vi "Do.vi"(8 "error in (no error)":errorcluster, 10 "Actor in":refnum<class "Actor.lvclass">, 11 "After Launch Init Msg":refnum<class "After Launch Init Msg.lvclass">) -> (0 "error out":errorcluster, 2 "Actor out":refnum<class "Actor.lvclass">)   [LabVIEW 2015, in "CS++BaseActor.lvlib" / "After Launch Init Msg.lvclass"]
doc: "This VI delivers the message to the actor by calling the appropriate method(s) on the actor."
uses:
  After Launch Init Msg.lvclass
  <vilib>/ActorFramework/Actor/Actor.lvclass
  CS++BaseActor/CS++BaseActor.lvclass
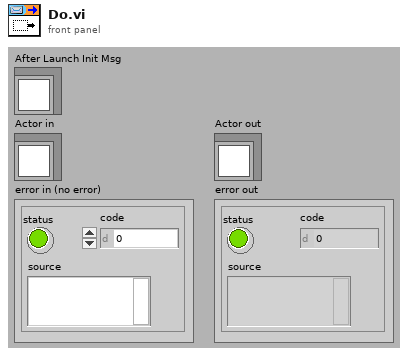
[diagram p1: front panel]
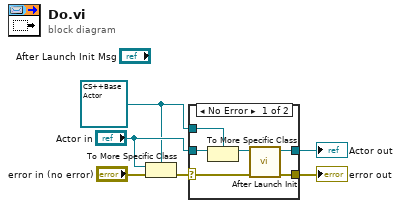
[diagram p0: block diagram]
diagram:
  w1 = refnum<class "CS++BaseActor.lvclass"> refnum ("Actor in")
  n1 = To More Specific Class(target class=w1, reference="Actor in", error in="error in (no error)") -> (error out=w5:errorcluster)  [unwired: 1 out]
  n2 = case shown="No Error" w5 {
    selector: w5 -> [w10 w14]
    tunnel: [w12 w14] -> w4
    tunnel: [w11 w13] -> w3
    tunnel: "Actor in" -> [w9 w13]
    tunnel: w1 -> [w8 _]
    frame No Error {
      n3 = To More Specific Class(target class=w8, reference=w9) -> (specific class reference=w7:refnum<class "CS++BaseActor.lvclass">)  [unwired: 1 in, 1 out]
      n4 = call "After Launch Init.vi"("error in (no error)"=w10, "CS++BaseActor in"=w7) -> ("error out"=w12:errorcluster, "CS++BaseActor out"=w11:refnum<class "CS++BaseActor.lvclass">)  [unwired: 8 in]
    }
    frame Error {
    }
  }
  "error out" <- w4
  "Actor out" <- w3
